vi "Append (SubVI).vi"(8 "error in (no error)":errorcluster, 10 "read buffer":string, 11 "file (use dialog)":path) -> (0 "error out":errorcluster)   [LabVIEW 2019]
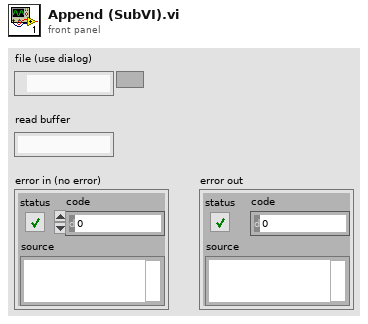
[diagram p1: front panel]
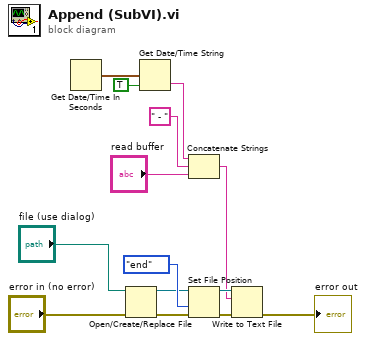
[diagram p0: block diagram]
diagram:
  n1 = Get Date/Time In Seconds() -> (seconds since 1Jan1904=w5:timestamp)
  n2 = Open/Create/Replace File(file path (use dialog)="file (use dialog)", error in="error in (no error)") -> (refnum out=w9:refnum<file>, error out=w8:errorcluster)  [unwired: 4 in, 1 out]
  n3 = Get Date/Time String(seconds (now)=w5, want seconds? (F)=TRUE) -> (time string=w3:string)  [unwired: 1 in, 1 out]
  n4 = Concatenate Strings(w3, " - " ("string"), "read buffer") -> (w1:string)
  n5 = Set File Position(refnum=w9, from (0:start)=enum16{"start", "end", "current"}."end", error in=w8) -> (refnum out=w14:refnum<file>, error out=w12:errorcluster)  [unwired: 1 in]
  n6 = Write to Text File(file (use dialog)=w14, text=w1, error in=w12) -> (error out=→"error out":errorcluster)  [unwired: 1 in, 2 out]
